vi "strip word.vi"() -> ()   [LabVIEW 2020]
panel:
  in  "energy fxp":fxp<+/-,16,1>
  out "hi(x) 2":u16
  out "hi(x)":u8
  out "lo(x)":u32 format="%b"
  out "(hi.lo)":u64 format="%b"
  in  "m 3":u8 format="%b"
  in  "m 2":u8 format="%b"
  in  "m 1":u8 format="%b"
  out "energy":i16
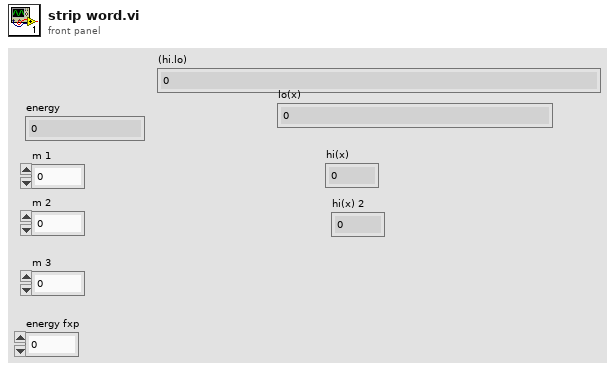
[diagram p1: front panel]
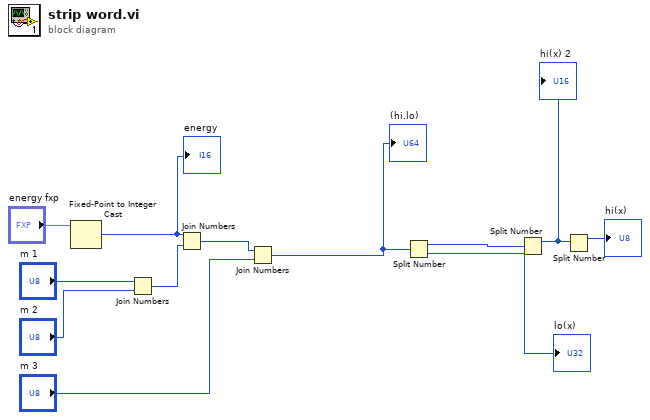
[diagram p0: block diagram]
diagram:
  n1 = Fixed-Point to Integer Cast(1:"energy fxp") -> (0:w2:i16)
  "energy" <- w2
  n2 = Join Numbers(hi="m 1", lo="m 2") -> ((hi.lo)=w10:u16)
  n3 = Join Numbers(hi=w2, lo=w10) -> ((hi.lo)=w9:u32)
  n4 = Join Numbers(hi=w9, lo="m 3") -> ((hi.lo)=w7:u64)
  "(hi.lo)" <- w7
  n5 = Split Number(x=w7) -> (hi(x)=w5:u32, lo(x)=→"lo(x)":u32)
  n6 = Split Number(x=w5) -> (hi(x)=w4:u16)  [unwired: 1 out]
  "hi(x) 2" <- w4
  n7 = Split Number(x=w4) -> (hi(x)=→"hi(x)":u8)  [unwired: 1 out]
